vi "Write.vi"(0 "element":bool) -> (1 "previous element":bool, 2 "channel":T1)   [LabVIEW 2020, in "Tag-bool.lvlib"]
doc: "Writes a value to a Tag channel."
uses:
  <extravilib>/ChannelInstances/Tag-bool.lvlib
  <extravilib>/ChannelInstances/Tag-bool/))Channel.ctl
  <extravilib>/ChannelInstances/Tag-bool/Endpoint.vi
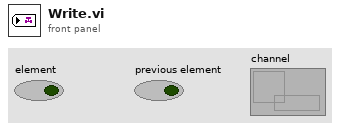
[diagram p1: front panel]
types:
  T1 = typedef "Tag-bool.lvlib/))Channel.ctl" = refnum<queue>
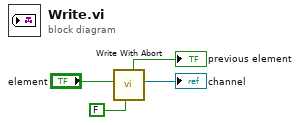
[diagram p0: block diagram]
diagram:
  n1 = call <extravilib>:"Write With Abort.vi"("abort"=FALSE, "element"="element") -> ("channel"=→"channel":T1, "previous element"=→"previous element":bool)  [unwired: 7 in, 1 out]
